vi "Handle Error.vi"(8 "error in (no error)":errorcluster, 11 "KIT-QVA in":refnum<class "KIT-QVA.lvclass">) -> (0 "error out":errorcluster, 2 "stop actor?":bool=TRUE, 3 "KIT-QVA out":refnum<class "KIT-QVA.lvclass">)   [LabVIEW 2014, in "KIT-QVA.lvlib" / "KIT-QVA.lvclass"]
doc: "(<B>Filename</B>: Actor Framework.lvlib:Actor.lvclass:Handle Error.vi)\n\nDefines how the actor handles an error that occurred while processing a message.\n\nBy default, this method does nothing except stop the actor. This method also treats error code 43 (coming from <B>error in</B>) as a sign that the actor shut down normally. In this situation, the Handle Error method does not return the error on <B>error out</B>, meaning the actor's caller will not receive it. All other error codes will be returned on <B>error out</B>.\n\nA descendant class may override this method to change this behavior."
uses:
  KIT-QVA.lvclass
  CSPP_Core/Actors/CS++BaseActor/CS++BaseActor.lvclass/CS++BaseActor.ctl
  CSPP_Core/Actors/CS++DeviceActor/CS++DeviceActor.lvclass/CS++DeviceActor.ctl
  <vilib>/ActorFramework/Actor/Actor.lvclass/Actor.ctl
  <vilib>/ActorFramework/Message Enqueuer/Message Enqueuer.lvclass/Message Enqueuer.ctl
  CSPP_Core/Actors/CS++DeviceActor Messages/Initialize Device Msg/Initialize Device Msg.lvclass/Initialize Device Msg.ctl
  <vilib>/ActorFramework/Message Enqueuer/Init from Existing Queue.vi
  <vilib>/ActorFramework/Message Enqueuer/Enqueue.vi
  <vilib>/ActorFramework/Message Priority Queue/Priority Enqueue.vi
  CSPP_Core/Actors/CS++DeviceActor/CS++DeviceActor.lvclass
  CSPP_Core/Actors/CS++DeviceActor Messages/Initialize Device Msg/Initialize Device Msg.lvclass
  <vilib>/ActorFramework/Message Enqueuer/Message Enqueuer.lvclass
  <vilib>/ActorFramework/Actor/Actor.lvclass
  CSPP_Core/Libraries/Utilities/CS++Utilities.lvlib
  CSPP_Core/Actors/CS++BaseActor/CS++BaseActor.lvclass
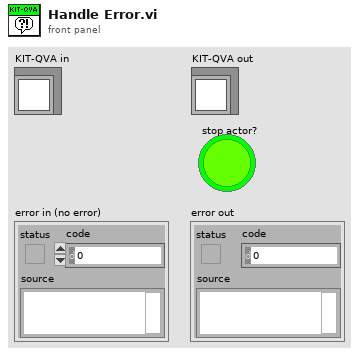
[diagram p1: front panel]
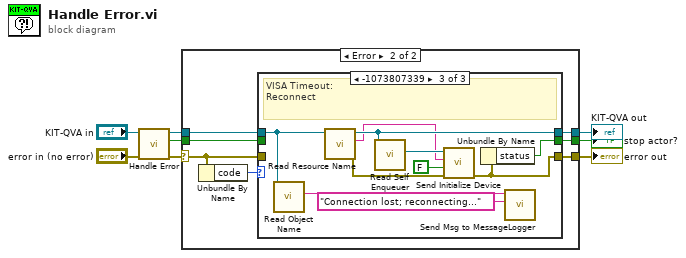
[diagram p0: block diagram]
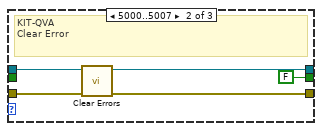
[diagram p4: hidden frame]
diagram:
  n1 = call-parent "Handle Error.vi"("error in (no error)"="error in (no error)", "CS++DeviceActor in"="KIT-QVA in") -> ("error out"=w6:errorcluster, "stop actor?"=w3:bool, "CS++DeviceActor out"=w2:refnum<class "KIT-QVA.lvclass">)  [unwired: 7 in]
  n2 = case shown="Error" w6 {
    selector: w6 -> [w11 w12]
    tunnel: [w11 w13] -> w5
    tunnel: [w10 w15] -> w4
    tunnel: w3 -> [w10 w14]
    tunnel: w2 -> [w9 w16]
    tunnel: [w9 w17] -> w1
    frame No Error {
    }
    frame Error {
      n3 = Unbundle By Name(w12) -> ("code"=w18:i32)
      n4 = case shown="-1073807339" w18 {
        tunnel: [w21 w25 w35] -> w17
        tunnel: w16 -> [w21 w25 w28]
        tunnel: [w20 FALSE ("stop actor?") w30] -> w15
        tunnel: w14 -> [w20 _ _]
        tunnel: [w19 w22 w31] -> w13
        tunnel: w12 -> [w19 w24 _]
        frame Default {
        }
        frame 5000..5007 {
          # "KIT-QVA\nClear Error"
          n5 = call <vilib>:"Clear Errors.vi"("error in (no error)"=w24) -> ("error out"=w22:errorcluster)  [unwired: 5 in, 1 out]
        }
        frame -1073807339 {
          # "VISA Timeout:\nReconnect"
          n6 = call "Read Object Name.vi"("CS++BaseActor in"=w28) -> ("Object Name"=w27:string)  [unwired: 8 in, 2 out]
          n7 = call "Read Resource Name.vi"("CS++DeviceActor in"=w28) -> ("error out"=w29:errorcluster, "Resource Name"=w33:string, "CS++DeviceActor out"=w35:refnum<class "KIT-QVA.lvclass">)  [unwired: 8 in]
          n8 = call <vilib>:"Read Self Enqueuer.vi"("Actor"=w35) -> ("Self Enqueuer"=w34:refnum<class "Message Enqueuer.lvclass">)  [unwired: 10 in]
          n9 = call "Send Initialize Device.vi"("error in (no error)"=w29, "Reset (F)"=FALSE, "Resource Name"=w33, "Message Enqueuer"=w34) -> ("error out"=w31:errorcluster)  [unwired: 6 in, 1 out]
          n10 = Unbundle By Name(w31) -> ("status"=w30:bool)
          n11 = call "Send Msg to MessageLogger.vi"("Message Content"="Connection lost; reconnecting...", "Message Tag"=w27) -> ()  [unwired: 9 in, 1 out]
        }
      }
    }
  }
  "KIT-QVA out" <- w1
  "error out" <- w5
  "stop actor?" <- w4
